vi "macro_SwerveDrivePoseEst2_Execute.vi"() -> ()   [LabVIEW 2019, in "Trajectory_Library.lvlib"]
uses:
  TypeDef/POSE2D.ctl
  TypeDef/TRANSLATION2D.ctl
  TypeDef/ROTATION2D.ctl
  VI/Util_GetTime_U32.vi
  VI/Util_GetTime_U64.vi
  Trajectory_Library.lvlib
  TypeDef/SWERVE_DRIVE_MODULE_POSITION.ctl
panel:
  in  "Module Positions":T1[](array[typedef]) {"Angle"."SIN" format="%13.4f"; "Angle"."COS" format="%13.4f"; "Angle"."VALUE" format="%13.4f"}
  in  "Vision TImeStamp_Seconds":dbl=0.02
  in  "visionRobotPose":T3={"TRANSLATION"={"X"=0.0, "Y"=0.0}, "ROTATION"={"VALUE"=0.0, "COS"=1.0, "SIN"=0.0}} {"ROTATION"."SIN" format="%13.4f"; "ROTATION"."COS" format="%13.4f"; "ROTATION"."VALUE" format="%13.4f"; "TRANSLATION"."Y" format="%14.3f"; "TRANSLATION"."X" format="%14.3f"}
  in  "Add Vision Meas":bool
  in  "Game Started":bool=TRUE
  in  "InitialPose":T3={"TRANSLATION"={"X"=0.0, "Y"=0.0}, "ROTATION"={"VALUE"=0.0, "COS"=1.0, "SIN"=0.0}} {"ROTATION"."SIN" format="%13.4f"; "ROTATION"."COS" format="%13.4f"; "ROTATION"."VALUE" format="%13.4f"; "TRANSLATION"."Y" format="%14.3f"; "TRANSLATION"."X" format="%14.3f"}
  in  "Gyro Degrees":dbl
  out "Estimated Pose":T3={"TRANSLATION"={"X"=0.0, "Y"=0.0}, "ROTATION"={"VALUE"=0.0, "COS"=1.0, "SIN"=0.0}} {"ROTATION"."SIN" format="%13.4f"; "ROTATION"."COS" format="%13.4f"; "ROTATION"."VALUE" format="%13.4f"; "TRANSLATION"."Y" format="%14.3f"; "TRANSLATION"."X" format="%14.3f"}
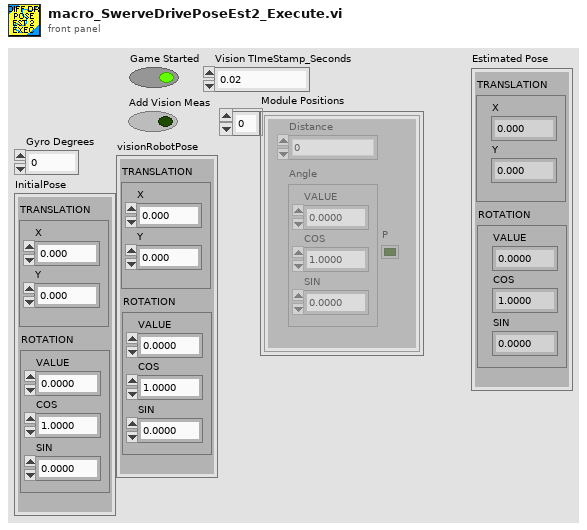
[diagram p1: front panel]
types:
  T1 = typedef "Trajectory_Library.lvlib/SWERVE_DRIVE_MODULE_POSITION.ctl" = cluster{"Distance":dbl, "Angle":T2, "P":bool}
  T2 = typedef "Trajectory_Library.lvlib/ROTATION2D.ctl" = cluster{"VALUE":dbl, "COS":dbl, "SIN":dbl}
  T3 = typedef "Trajectory_Library.lvlib/POSE2D.ctl" = cluster{"TRANSLATION":T4, "ROTATION":T2}
  T4 = typedef "Trajectory_Library.lvlib/TRANSLATION2D.ctl" = cluster{"X":dbl, "Y":dbl}
  T5 = typedef "Trajectory_Library.lvlib/SWERVE_DRIVE_POSE_EST2_CONFIG.ctl" = cluster{"Wheel_Locations M":T4[], "Odom X std dev M":dbl, "Odom Y std dev M":dbl, "Odom Heading std dev Rad":dbl, "Vision X std dev M":dbl, "Vision Y std dev M":dbl, "Vision Heading std dev Rad":dbl}
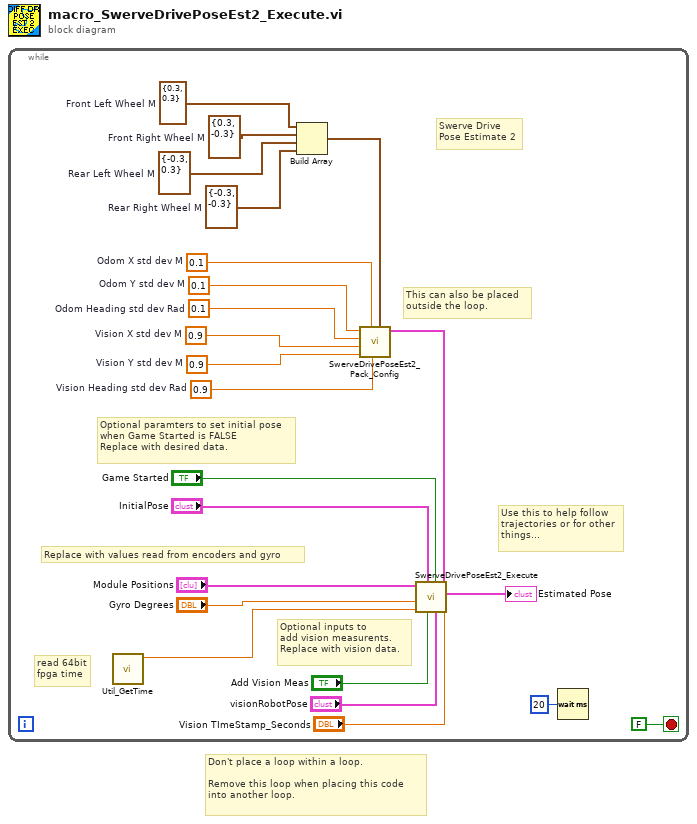
[diagram p0: block diagram]
diagram:
  # "Don't place a loop within a loop.\n \nRemove this loop when placing this code\ninto another loop."
  n1 = while {
    stop <- FALSE stop-if-true
    w3 = T4 {"X"=-0.3, "Y"=-0.3}  # Rear Right Wheel M
    w4 = T4 {"X"=-0.3, "Y"=0.3}  # Rear Left Wheel M
    w5 = T4 {"X"=0.3, "Y"=-0.3}  # Front Right Wheel M
    w6 = T4 {"X"=0.3, "Y"=0.3}  # Front Left Wheel M
    w16 = 0.1  # Odom Y std dev M
    w17 = 0.1  # Odom Heading std dev Rad
    w18 = 0.9  # Vision X std dev M
    w19 = 0.9  # Vision Y std dev M
    w20 = 0.1  # Odom X std dev M
    w21 = 0.9  # Vision Heading std dev Rad
    # "Optional inputs to\nadd vision measurents.\nReplace with vision data."
    # "Replace with values read from encoders and gyro"
    # "Optional paramters to set initial pose\nwhen Game Started is FALSE\nReplace with desired data."
    # "read 64bit\nfpga time"
    # "This can also be placed \noutside the loop."
    # "Use this to help follow\ntrajectories or for other\nthings..."
    # "Swerve Drive \nPose Estimate 2"
    n2 = call "Util_GetTime.vi"() -> ("FPGA_Time_Seconds"=w13:dbl)  [unwired: 9 in, 2 out]
    n3 = Build Array(w6, w5, w4, w3) -> (w2:T4[])
    n4 = call "SwerveDrivePoseEst2_Pack_Config.vi"("Wheel_Locations M"=w2, "Vision Heading std dev Rad"=w21, "Odom X std dev M"=w20, "Vision Y std dev M"=w19, "Vision X std dev M"=w18, "Odom Heading std dev Rad"=w17, "Odom Y std dev M"=w16) -> ("SwervePoseEst2Config"=w7:T5)  [unwired: 4 in]
    n5 = call "SwerveDrivePoseEst2_Execute.vi"("Vision TImeStamp_Seconds"="Vision TImeStamp_Seconds", "SwervePoseEst2Config"=w7, "visionRobotPose"="visionRobotPose", "Game Started"="Game Started", "Add Vision Meas"="Add Vision Meas", "InitialPose"="InitialPose", "Pass Through Time"=w13, "Gyro Degrees"="Gyro Degrees", "Module Positions"="Module Positions") -> ("Estimated Pose"=→"Estimated Pose":T3)  [unwired: 1 in, 1 out]
    n6 = Wait (ms)(milliseconds to wait=u32 20) -> ()  [unwired: 1 out]
  }
